vi "Submit Ingestion Config.vi"(8 "error in (no error)":errorcluster, 10 "Asset Name":string, 11 "Sift Client in":refnum<class "Sift Client.lvclass">) -> (0 "error out":errorcluster, 2 "Ingestion Config ID":string, 3 "Sift Client out":refnum<class "Sift Client.lvclass">)   [LabVIEW 2024, in "Sift Client.lvlib" / "Sift Client.lvclass"]
doc: "Submit the ingestion config to Sift. Only call this after all channels and flows have been registered."
uses:
  Sift Client.lvclass
  Private/Typedefs/Ingestion Config/Ingestion Config.ctl
  Private/Typedefs/Ingestion Config/Flow Config.ctl
  Private/Typedefs/Ingestion Config/Channel Config.ctl
  Types/Data Type.ctl
  Types/Bit Field.ctl
  Types/Enum.ctl
  Private/Typedefs/Messages/JSON Request.ctl
  Private/Typedefs/Messages/Create Ingestion Config Response.ctl
  Sift Client.lvclass/Sift Client.ctl
  <vilib>/Utility/error.llb/Error Cluster From Error Code.vi
  <vilib>/ErrorRing/Error Ring.xnode
  Sift Client.lvlib
  <vilib>/addons/_JKI.lib/Serialization/JSON/JKI JSON Serialization.lvlib
  <userlib>/_OpenG.lib/error/error.llb/openg_error.lvlib
panel:
  in  "Create Ingestion Config Reponse":T1
  in  "JSON Request":T2
  in  "Ingestion Config":T3
  out "JSON String":string
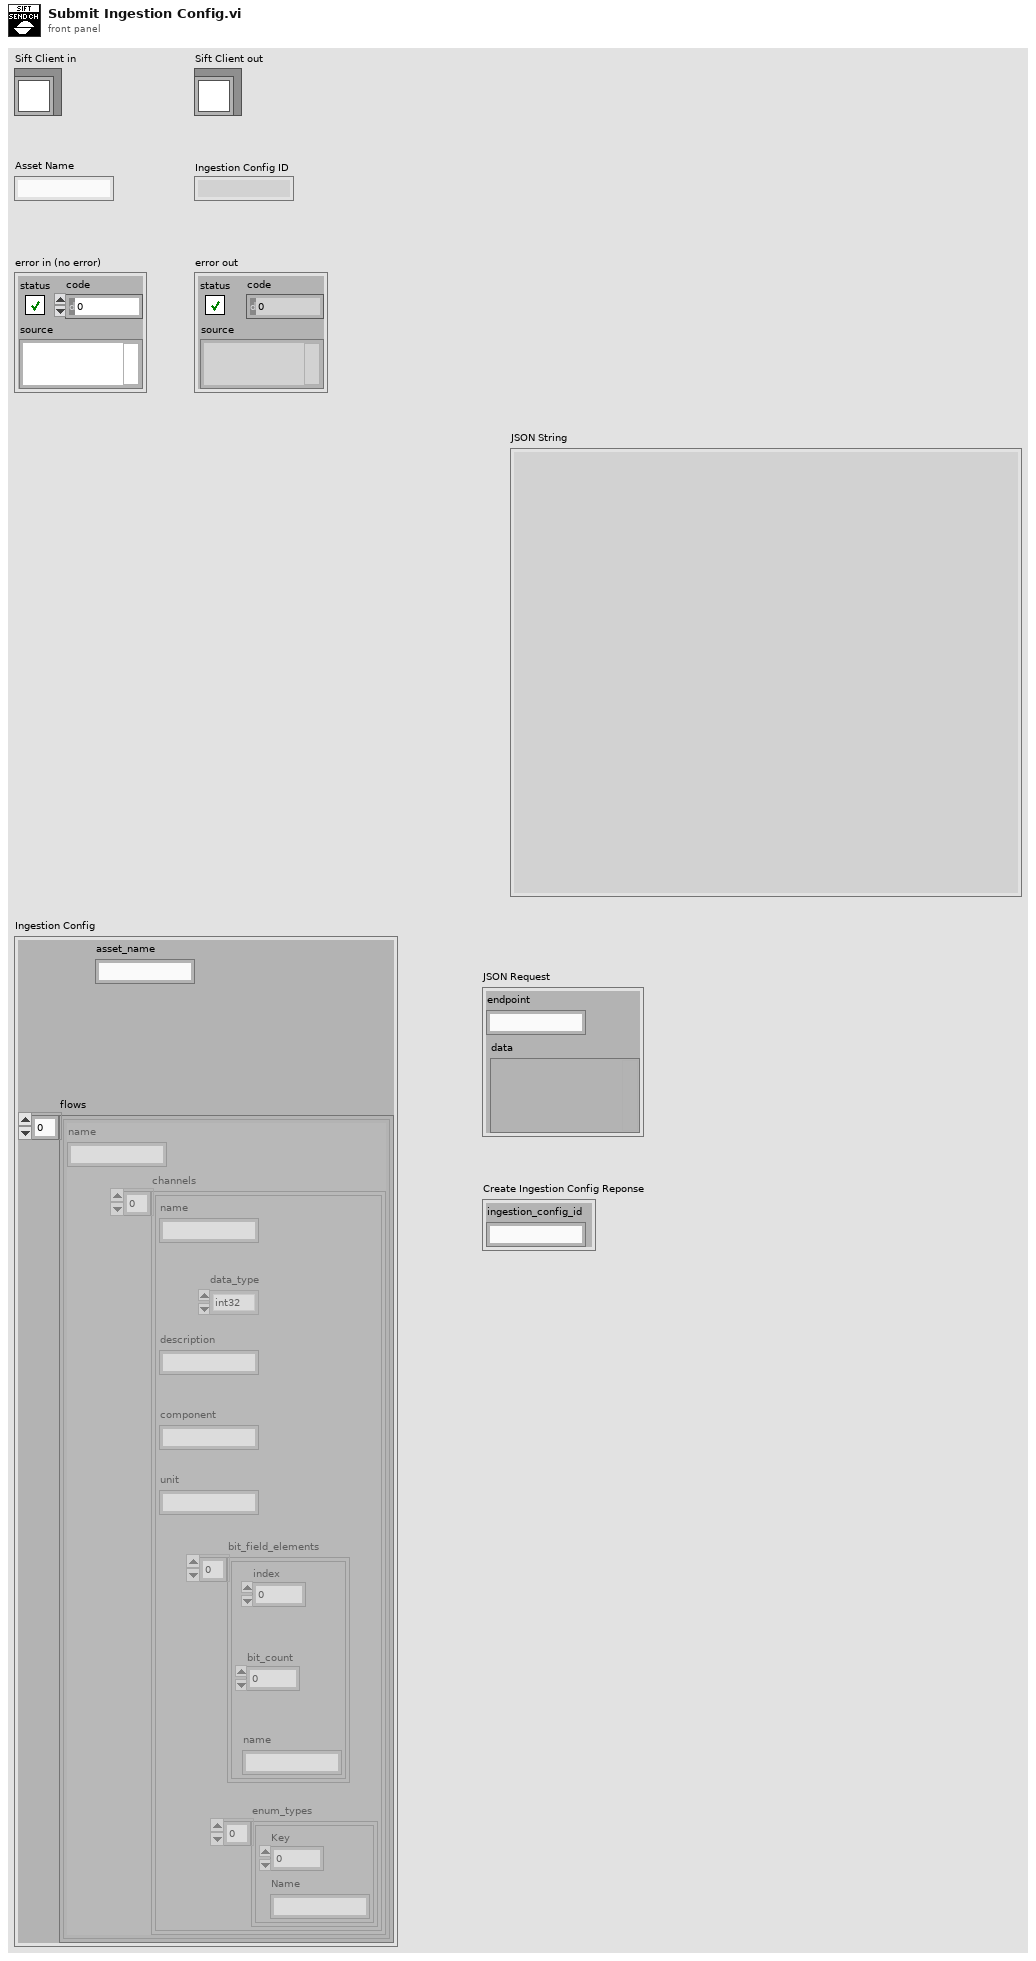
[diagram p1: front panel]
types:
  T1 = typedef "Sift Client.lvlib/Create Ingestion Config Response.ctl" = cluster{"ingestion_config_id":string}
  T2 = typedef "Sift Client.lvlib/JSON Request.ctl" = cluster{"endpoint":string, "data":variant}
  T3 = typedef "Sift Client.lvlib/Ingestion Config.ctl" = cluster{"asset_name":string, "flows":T4[]}
  T4 = typedef "Sift Client.lvlib/Flow Config.ctl" = cluster{"name":string, "channels":T5[]}
  T5 = typedef "Sift Client.lvlib/Channel Config.ctl" = cluster{"name":string, "data_type":T6, "description":string, "component":string, "unit":string, "bit_field_elements":T7[], "enum_types":T8[]}
  T6 = typedef "Sift Client.lvlib/Data Type.ctl" = enum8{"double", "float", "uint64", "int64", "uint32", "int32", "bool", "bit field", "enum"}
  T7 = typedef "Sift Client.lvlib/Bit Field.ctl" = cluster{"index":u32, "bit_count":u32, "name":string}
  T8 = typedef "Sift Client.lvlib/Enum.ctl" = cluster{"Key":u32, "Name":string}
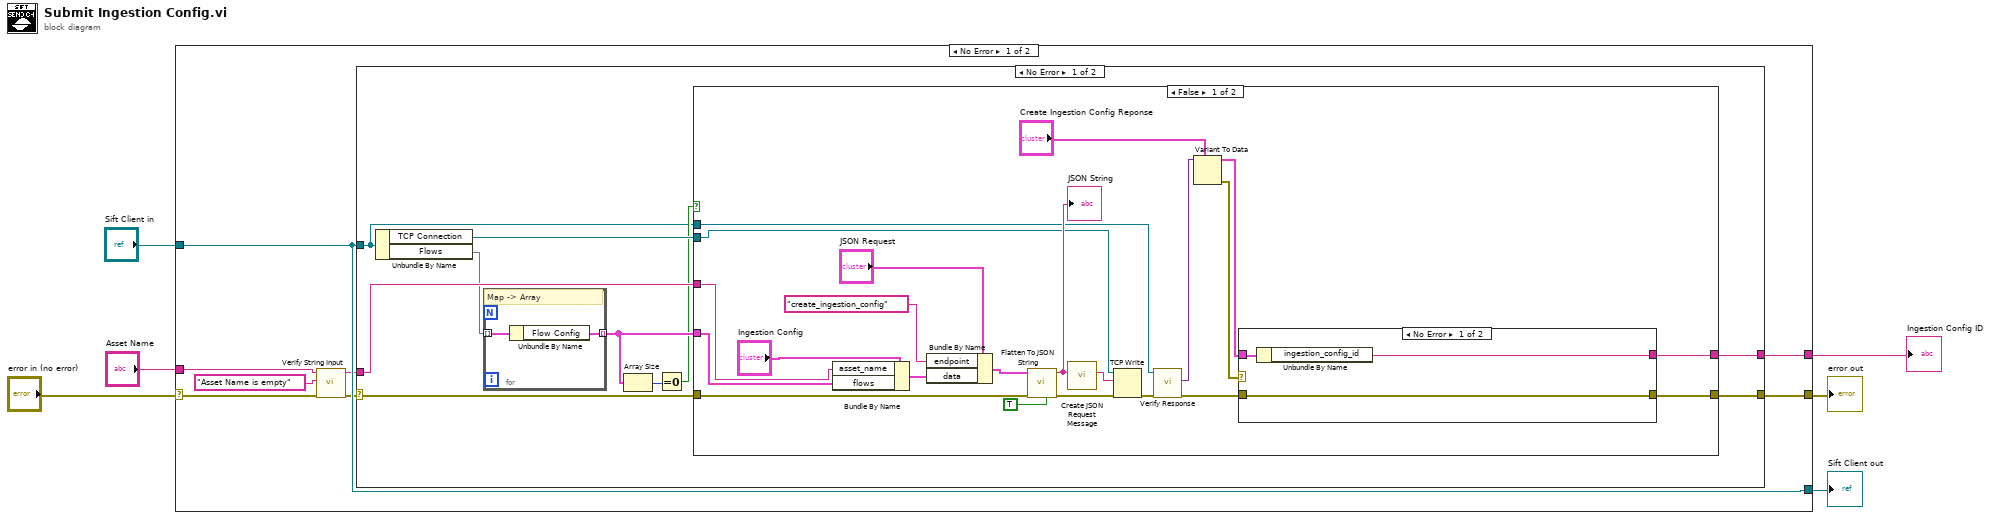
[diagram p0: block diagram]
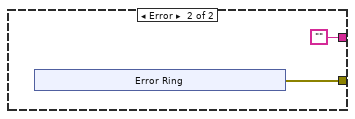
[diagram p2: hidden frame]
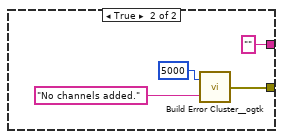
[diagram p3: hidden frame]
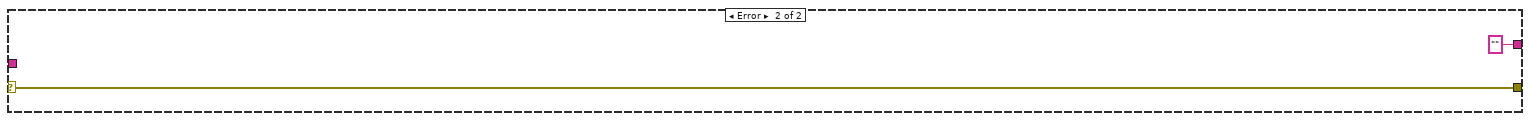
[diagram p4: hidden frame]
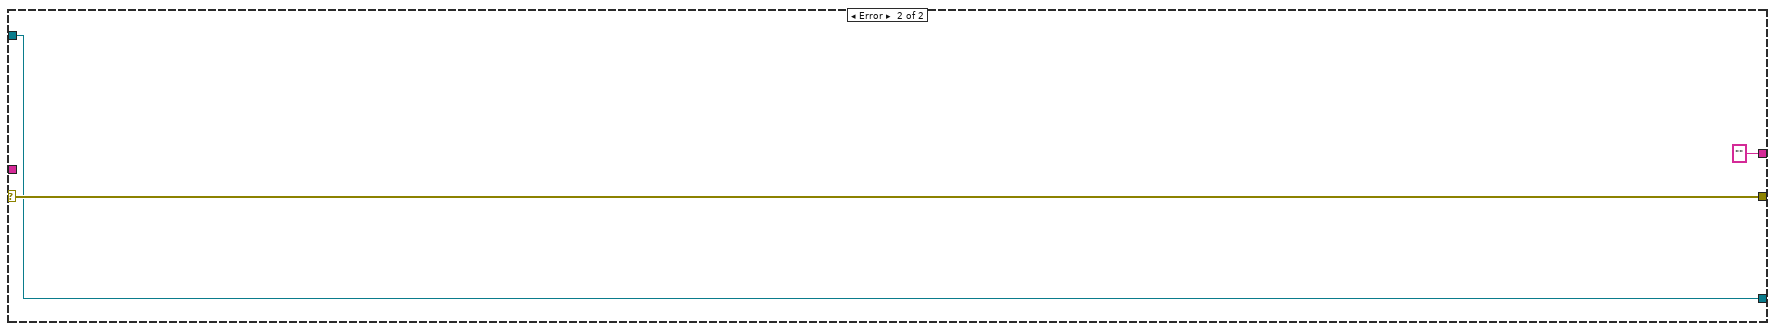
[diagram p5: hidden frame]
diagram:
  n1 = case shown="No Error" "error in (no error)" {
    selector: "error in (no error)" -> [w10 w67]
    tunnel: [w14 w67] -> w5
    tunnel: [w13 w66] -> w3
    tunnel: "Sift Client in" -> [w13 w66]
    tunnel: "Asset Name" -> [w12 _]
    tunnel: [w7 "" ("ingestion_config_id")] -> w1
    frame No Error {
      n2 = call "Verify String Input.vi"("error in (no error)"=w10, "Error Message"="Asset Name is empty", "Input"=w12) -> ("error out"=w8:errorcluster, "Output"=w9:string)  [unwired: 7 in]
      n3 = case shown="No Error" w8 {
        selector: w8 -> [w17 w64]
        tunnel: [w23 w64] -> w14
        tunnel: w13 -> [w16 _]
        tunnel: w9 -> [w22 _]
        tunnel: [w15 "" ("ingestion_config_id")] -> w7
        frame No Error {
          n4 = Unbundle By Name(w16) -> ("TCP Connection"=w24:refnum<k5>, "Flows"=w21:map{string, T4})
          n5 = for {
            tunnel: [w25] -> w20 mode=indexing
            tunnel: w21 -> [w26] mode=indexing
            # "Map -> Array"
            n6 = Unbundle By Name(w26) -> ("Flow Config"=w25:T4)
          }
          n7 = Array Size(array=w20) -> (size(s)=w19:i32)
          n8 = Equal To 0?(x=w19) -> (x = 0?=w18:bool)
          n9 = case shown="False" w18 {
            tunnel: w22 -> [w46 _]
            tunnel: w24 -> [w43 _]
            tunnel: w17 -> [w48 _]
            tunnel: [w31 w60] -> w23
            tunnel: w20 -> [w45 _]
            tunnel: w16 -> [w39 _]
            tunnel: [w32 "" ("ingestion_config_id")] -> w15
            frame False {
              n10 = Bundle By Name(cluster="Ingestion Config", "asset_name"=w46, "flows"=w45) -> (w36:T3)
              n11 = Bundle By Name(cluster="JSON Request", "endpoint"="create_ingestion_config", "data"=w36) -> (w35:T2)
              n12 = call <vilib>:"Flatten To JSON String.vi"("Enums As String (F)"=TRUE, "error in"=w48, "Variant"=w35) -> ("error out"=w41:errorcluster, "JSON String"=w44:string)  [unwired: 7 in]
              "JSON String" <- w44
              n13 = call "Create JSON Request Message.vi"("Data"=w44) -> ("Message"=w42:string)  [unwired: 10 in]
              n14 = TCP Write(connection ID=w43, data in=w42, error in (no error)=w41) -> (error out=w38:errorcluster)  [unwired: 1 in, 2 out]
              n15 = call-dynamic "Verify Response.vi"("error in (no error)"=w38, "Sift Client in"=w39) -> ("error out"=w33:errorcluster, "data"=w30:variant)  [unwired: 7 in, 1 out]
              n16 = Variant To Data(type="Create Ingestion Config Reponse", Variant=w30) -> (data=w27:T1, error out=w28:errorcluster)  [unwired: 1 in]
              n17 = case shown="No Error" w28 {
                tunnel: [w49 ""] -> w32
                tunnel: [w51 w53] -> w31
                tunnel: w33 -> [w51 _]
                tunnel: w27 -> [w50 _]
                frame No Error {
                  n18 = Unbundle By Name(w50) -> ("ingestion_config_id"=w49:string)
                }
                frame Error {
                  n19 = xnode "Error Ring"() -> ("error out"=w53:errorcluster)
                }
              }
            }
            frame True {
              n20 = call <userlib>:"Build Error Cluster__ogtk.vi"("String to Prepend to source (\"\")"="No channels added." ("String to Prepend to source (\"\")"), "code"=5000) -> ("error out"=w60:errorcluster)
            }
          }
        }
        frame Error {
        }
      }
    }
    frame Error {
    }
  }
  "error out" <- w5
  "Sift Client out" <- w3
  "Ingestion Config ID" <- w1
